vi "Stabilize and Measure.vi"(8 "error in":errorcluster, 9 "Dont wait for Stabilization":bool=TRUE, 11 "Time between\nmeasurements (s)":dbl=2.0) -> (0 "error out":errorcluster, 1 "Data Cluster":T1, 2 "Waveforms":T5)   [LabVIEW 2013]
uses:
  Controls/arranged waveforms.ctl
  Controls/waveform display.ctl
  Controls/Data Cluster.ctl
  Controls/Power Values.ctl
  <vilib>/addons/Electrical Power/Basic/Measurement/subVIs/basic_Power Value.ctl
  Controls/Stabilization.ctl
  <vilib>/addons/Electrical Power/Basic/NI_EP_Basic.lvlib
panel:
  out "Stabilization Elapsed \nTime (min)":dbl format="%#_3g"
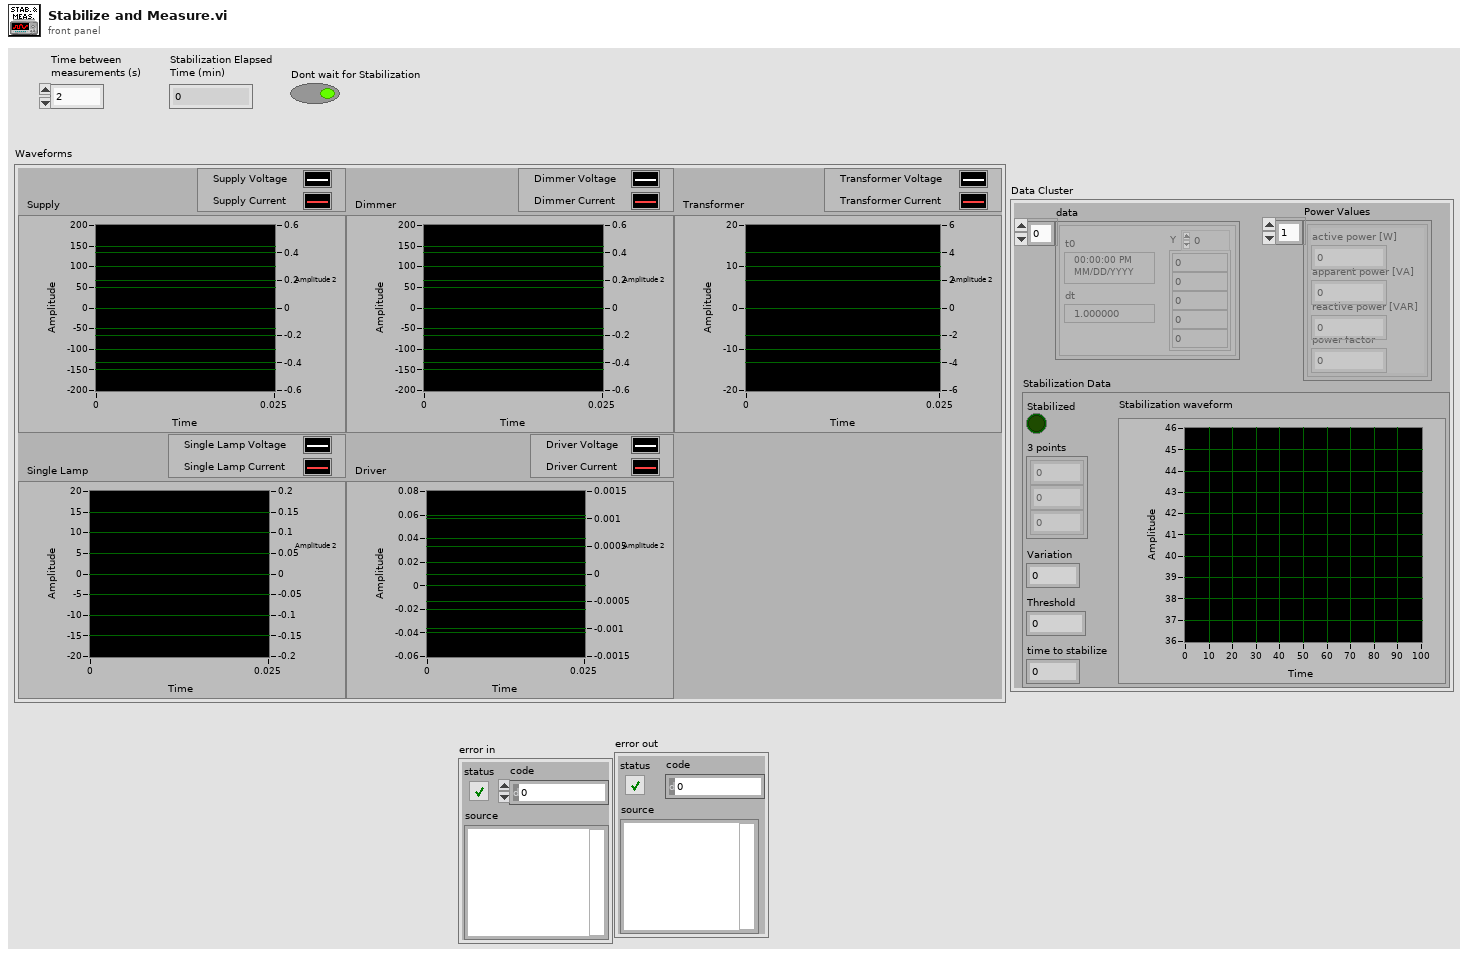
[diagram p1: front panel]
types:
  T1 = typedef "Data Cluster.ctl" = cluster{"data":waveform(dbl)[], "Power Values":T2, "Stabilization Data":T4}
  T2 = typedef "Power Values.ctl" = T3[]
  T3 = typedef "NI_EP_Basic.lvlib/basic_Power Value.ctl" = cluster{"active power [W]":dbl, "apparent power [VA]":dbl, "reactive power [VAR]":dbl, "power factor":dbl}
  T4 = typedef "Stabilization.ctl" = cluster{"Stabilization waveform":waveform(dbl), "Variation":dbl, "Stabilized":bool, "Threshold":dbl, "time to stabilize":dbl, "3 points":dbl[]}
  T5 = typedef "arranged waveforms.ctl" = cluster{"Supply":T6, "Dimmer":T6, "Transformer":T6, "Single Lamp":T6, "Driver":T6}
  T6 = typedef "waveform display.ctl" = waveform(dbl)[]
  T7 = cluster{"task out":refnum<k21>, "task out":refnum<k21>}
  T8 = cluster{"Refnum in":refnum<k21>, "Refnum in 2":refnum<k21>}
  T9 = cluster{"data":waveform(dbl)[], "Power Values":T2, "Stabilization Data":T4}
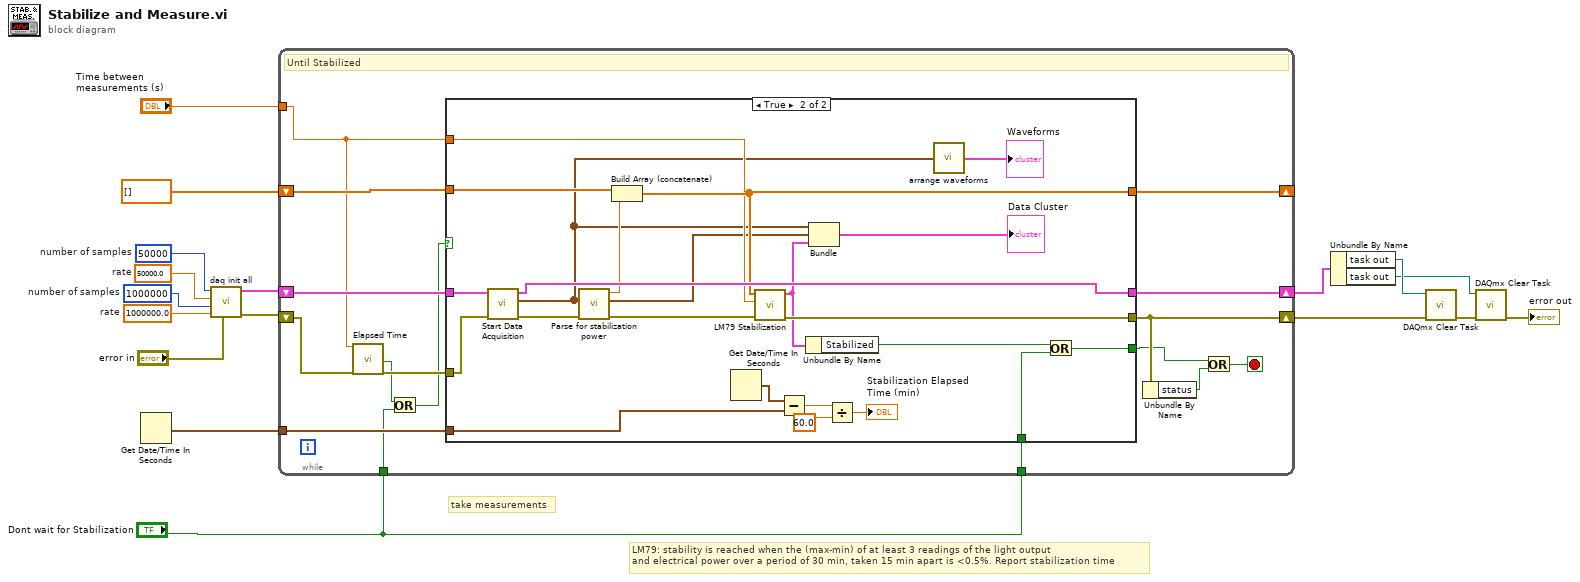
[diagram p0: block diagram]
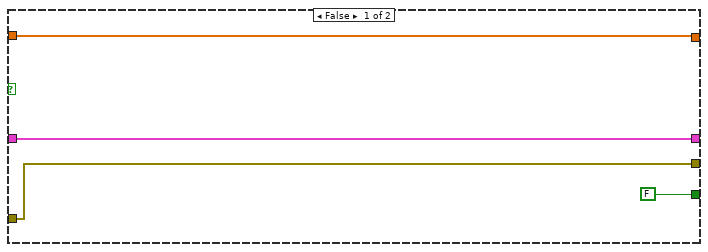
[diagram p2: hidden frame]
diagram:
  w1 = 1000000.0  # rate
  w2 = 1000000  # number of samples
  w3 = 50000.0  # rate
  w4 = 50000  # number of samples
  # "take measurements"
  # "LM79: stability is reached when the (max-min) of at least 3 readings of the light output\nand electrical power over a period of 30 min, taken 15 min apart is <0.5%. Report stabilization time"
  n1 = Get Date/Time In Seconds() -> (seconds since 1Jan1904=w15:timestamp)
  n2 = call "daq init all.vi"("error in"="error in", "rate 2"=w1, "number of samples 2"=w2, "rate"=w3, "number of samples"=w4) -> ("error out"=w6:errorcluster, "output cluster"=w7:T7)  [unwired: 5 in]
  n3 = while {
    tunnel: "Time between\nmeasurements (s)" -> [w25]
    shift-right: [w33] -> w12
    shift-left: w7 -> [w32]
    shift-right: [w21] -> w16
    shift-left: w6 -> [w27]
    tunnel: "Dont wait for Stabilization" -> [w31]
    tunnel: w15 -> [w30]
    shift-right: [w28] -> _
    shift-left: dbl[] [] -> [w29]
    tunnel: "Dont wait for Stabilization" -> [w24]
    stop <- w18 stop-if-true
    # "Until Stabilized"
    n4 = call "Elapsed Time"("Time Target (s)"=w25, "error in (no error)"=w27) -> ("Time has Elapsed"=w23:bool, "error out"=w26:errorcluster)  [unwired: 10 in, 6 out]
    n5 = Or(x=w23, y=w24) -> (x .or. y?=w22:bool)
    n6 = case shown="True" w22 {
      tunnel: [w35 w60] -> w33
      tunnel: w32 -> [w35 w59]
      tunnel: [FALSE w58] -> w20
      tunnel: w31 -> [_ w57]
      tunnel: w30 -> [_ w55]
      tunnel: w29 -> [w34 w50]
      tunnel: [w34 w47] -> w28
      tunnel: w25 -> [_ w46]
      tunnel: [w37 w44] -> w21
      tunnel: w26 -> [w37 w43]
      frame False {
      }
      frame True {
        n7 = call "Start Data Acquisition.vi"("error in (no error)"=w43, "Cluster"=w59) -> ("error out"=w49:errorcluster, "data"=w38:waveform(dbl)[], "Cluster 2"=w60:T8)  [unwired: 7 in]
        n8 = call "Parse for stabilization power.vi"("error in (no error)"=w49, "data"=w38) -> ("error out"=w48:errorcluster, "Power Values"=w42:T2, "active power [W]"=w51:dbl)  [unwired: 7 in]
        n9 = Build Array (concatenate)(w50, w51) -> (w47:dbl[])
        n10 = Get Date/Time In Seconds() -> (seconds since 1Jan1904=w56:timestamp)
        n11 = call "LM79 Stabilization.vi"("error in (no error)"=w48, "Time Between\nMeasurements (ms)"=w46, "Data over time"=w47) -> ("error out"=w44:errorcluster, "Stabilization Data"=w41:T4)  [unwired: 7 in]
        n12 = Subtract(x=w56, y=w55) -> (x-y=w54:dbl)
        n13 = Unbundle By Name(w41) -> ("Stabilized"=w45:bool)
        n14 = Bundle("data"=w38, "Power Values"=w42, "Stabilization Data"=w41) -> (→"Data Cluster":T9)  [unwired: 1 in]
        n15 = Divide(x=w54, y=60.0) -> (x/y=→"Stabilization Elapsed \nTime (min)":dbl)
        n16 = call "arrange waveforms.vi"("data"=w38) -> ("Waveforms"=→"Waveforms":T5)
        n17 = Or(x=w45, y=w57) -> (x .or. y?=w58:bool)
      }
    }
    n18 = Unbundle By Name(w21) -> ("status"=w19:bool)
    n19 = Or(x=w20, y=w19) -> (x .or. y?=w18:bool)
  }
  n20 = Unbundle By Name(w12) -> ("task out"=w11:refnum<k21>, "task out"=w10:refnum<k21>)
  n21 = call <vilib>:"DAQmx Clear Task.vi"("task in"=w11, "error in"=w16) -> ("error out"=w9:errorcluster)  [unwired: 13 in]
  n22 = call <vilib>:"DAQmx Clear Task.vi"("task in"=w10, "error in"=w9) -> ("error out"=→"error out":errorcluster)  [unwired: 13 in]
